vi "SpeakerController.vi"(10 "SongWaveform":dbl[](array[numeric]), 11 "JoystickData":T1) -> (3 "Voltage":dbl)   [LabVIEW 2016]
doc: "Outputs the voltage to send to the speaker. When a button on the joystick is pressed, starts the music over."
uses:
  JoystickData/JoystickData.ctl
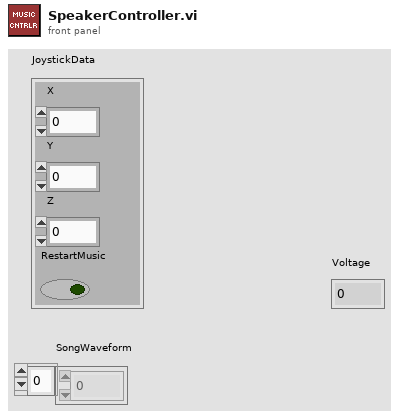
[diagram p1: front panel]
types:
  T1 = typedef "JoystickData.ctl" = cluster{"X":dbl, "Y":dbl, "Z":dbl, "RestartMusic":bool}
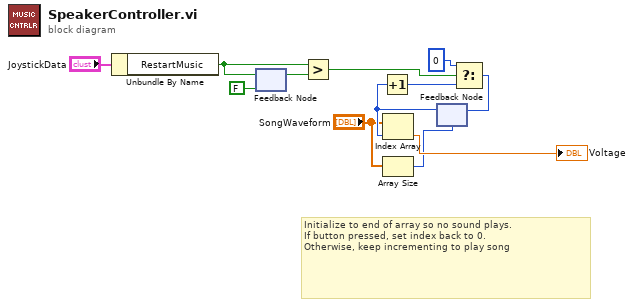
[diagram p0: block diagram]
diagram:
  # "Initialize to end of array so no sound plays.\nIf button pressed, set index back to 0.\nOtherwise, keep incrementing to play song"
  n1 = Unbundle By Name("JoystickData") -> ("RestartMusic"=w3:bool)
  n2 = feedback-in #1(w3) -> ()
  n3 = feedback #1(FALSE ("RestartMusic")) -> (w2:bool)
  n4 = Greater?(x=w3, y=w2) -> (0:w1:bool)
  n5 = Array Size(array="SongWaveform") -> (size(s)=w5:i32)
  n6 = feedback #2(w5) -> (w9:i32)
  n7 = Increment(x=w9) -> (x+1=w10:i32)
  n8 = Index Array(array="SongWaveform", index=w9) -> (element=→"Voltage":dbl)
  n9 = Select(t=0, s=w1, f=w10) -> (s? t:f=w7:i32)
  n10 = feedback-in #2(w7) -> ()
